vi "MotorOpenSynchronization.vi"(0 "error in (no error)":errorcluster, 5 "MotorData":T1[](array[typedef]), 6 "COM Port in":refnum<visa-resource-name>) -> (1 "Notifiers out":refnum<notifier>[](array[refnum]), 2 "Queue Reference out":refnum<notifier>[](array[refnum]), 3 "error out":errorcluster, 4 "Queue out":refnum<queue>, 8 "Queue name out":string, 9 "COM Port out":refnum<visa-resource-name>)   [LabVIEW 2009]
uses:
  Controls/MotorStatus.ctl
  Controls/MotorCommand.ctl
  Controls/MotorCommandBasic.ctl
  Controls/MotorData.ctl
  Controls/MotorNamedPosition.ctl
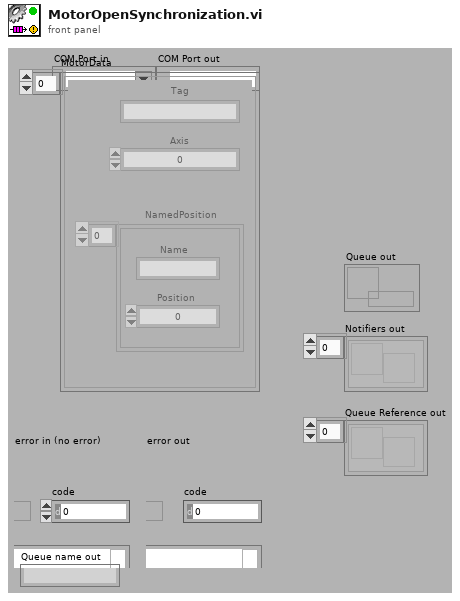
[diagram p1: front panel]
types:
  T1 = typedef "MotorData.ctl" = cluster{"Tag":string, "Axis":i32, "NamedPosition":T2[]}
  T2 = typedef "MotorNamedPosition.ctl" = cluster{"Position":i32, "Name":string}
  T3 = typedef "MotorCommand.ctl" = cluster{"Motor":string, "Command":T4, "Movement":i32, "Name":string, "Param":cluster{"VMIN":i32, "VMAX":i32, "ACC":i32}, "Ok?":refnum<k4>, "Go!":refnum<k4>}
  T4 = typedef "MotorCommandBasic.ctl" = enum16{"SELECT", "MOVE", "PREMOVE", "TURBO", "POS", "NAMED", "INIT", "STOP", "OFF", "SPEED", "QUIT"}
  T5 = typedef "MotorStatus.ctl" = cluster{"Managed?":bool, "Position":i32, "Name":string, "Status":enum16{"OFF", "IDLE", "MOVING", "HOMING"}}
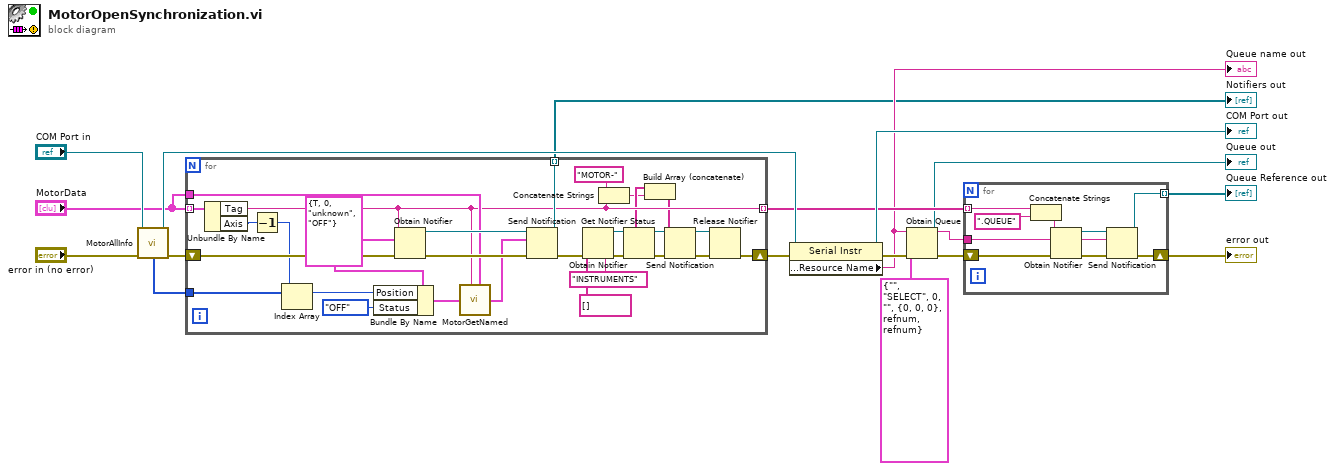
[diagram p0: block diagram]
diagram:
  n1 = call "MotorAllInfo.vi"("COM Port in"="COM Port in", "error in (no error)"="error in (no error)") -> ("COM Port out"=w11:refnum<visa-resource-name>, "Positions"=w14:i32[], "error out"=w15:errorcluster)  [unwired: 5 out]
  n2 = for {
    shift-right: [w30] -> w13
    shift-left: w15 -> [w46]
    tunnel: [w44] -> w4 mode=indexing
    tunnel: "MotorData" -> [w36] mode=indexing
    tunnel: w14 -> [w40]
    tunnel: [w31] -> w8 mode=indexing
    tunnel: "MotorData" -> [w35]
    w41 = T5 {"Managed?"=TRUE, "Position"=0, "Name"="unknown", "Status"=enum."OFF"} ("Axis Status")
    n3 = Unbundle By Name(w36) -> ("Tag"=w31:string, "Axis"=w38:i32)
    n4 = Decrement(x=w38) -> (x-1=w37:i32)
    n5 = Index Array(array=w40, index=w37) -> (element=w39:i32)
    n6 = Bundle By Name(cluster=w41, "Position"=w39, "Status"=enum16{"OFF", "IDLE", "MOVING", "HOMING"}."OFF") -> (w34:T5)
    n7 = Obtain Notifier(name (unnamed)=w31, notification data type=w41, error in (no error)=w46) -> (notifier out=w42:refnum<notifier>, error out=w45:errorcluster)  [unwired: 1 in, 1 out]
    n8 = call "MotorGetNamed.vi"("Motor status in"=w34, "MotorName"=w31, "MotorData"=w35) -> ("Motor status out"=w33:T5)
    n9 = Send Notification(notification=w33, notifier=w42, error in (no error)=w45) -> (notifier out=w44:refnum<notifier>, error out=w32:errorcluster)
    n10 = Obtain Notifier(name (unnamed)="INSTRUMENTS", notification data type=string[] [], error in (no error)=w32) -> (notifier out=w26:refnum<notifier>, error out=w27:errorcluster)  [unwired: 1 in, 1 out]
    n11 = Concatenate Strings("MOTOR-", w31) -> (w23:string)
    n12 = Get Notifier Status(notifier=w26, error in (no error)=w27) -> (notifier out=w19:refnum<notifier>, current notification=w25:string[], error out=w22:errorcluster)  [unwired: 2 out]
    n13 = Build Array (concatenate)(w25, w23) -> (w18:string[])
    n14 = Send Notification(notification=w18, notifier=w19, error in (no error)=w22) -> (notifier out=w20:refnum<notifier>, error out=w21:errorcluster)
    n15 = Release Notifier(notifier=w20, error in (no error)=w21) -> (error out=w30:errorcluster)  [unwired: 3 out]
  }
  "Notifiers out" <- w4
  n16 = property class="Serial Instr"(reference=w11, error in=w13) -> (reference out=→"COM Port out":refnum<visa-resource-name>, error out=w12:errorcluster, "General Settings:Resource Name"=w7:string)
  "Queue name out" <- w7
  n17 = Obtain Queue(name (unnamed)=w7, element data type=T3 {"Motor"="", "Command"=enum."SELECT", "Movement"=0, "Name"="", "Param"={"VMIN"=0, "VMAX"=0, "ACC"=0}, "Ok?"=refnum, "Go!"=refnum} ("MotorCommand"), error in (no error)=w12) -> (queue out=→"Queue out":refnum<queue>, error out=w9:errorcluster)  [unwired: 2 in, 1 out]
  n18 = for {
    shift-right: [w51] -> w5
    shift-left: w9 -> [w55]
    tunnel: [w53] -> w6 mode=indexing
    tunnel: w7 -> [w47]
    tunnel: w8 -> [w50] mode=indexing
    n19 = Concatenate Strings(w50, ".QUEUE") -> (w48:string)
    n20 = Obtain Notifier(name (unnamed)=w48, notification data type=w47, error in (no error)=w55) -> (notifier out=w52:refnum<notifier>, error out=w54:errorcluster)  [unwired: 1 in, 1 out]
    n21 = Send Notification(notification=w47, notifier=w52, error in (no error)=w54) -> (notifier out=w53:refnum<notifier>, error out=w51:errorcluster)
  }
  "error out" <- w5
  "Queue Reference out" <- w6
